vi "OFBS_displaySolution.vi"(7 "Results ListBox Ref":refnum<vi>, 8 "Stop Notifier In":refnum<notifier>, 9 "Control Refs":T1, 10 "Solution notifier":refnum<notifier>, 11 "BandGlobalOpt.lvclass":refnum<class "OptFreqBandsSearch.lvclass">) -> ()   [LabVIEW 2016, in "Optimal Frequency Bands Search.lvlib"]
doc: "Вывод текущего решения на экран. Оценка точности класификации (на тестовых данных). Обновление графиков приспособленности и точности классификации."
uses:
  GA_core/GA_tSolution progress.ctl
  OptFreqBandsSearch.lvclass
  OFBS_DataTypes.ctl
  Optimal Frequency Bands Search.lvlib
  GA_core/GeneticAlgorithm.lvlib
panel:
  # "This VI is a part of BCI Design library, http://www.ru-bci.org \nCopyright © 2020, Sotnikov Peter, All rights reserved. License: CC BY-NC 4.0"
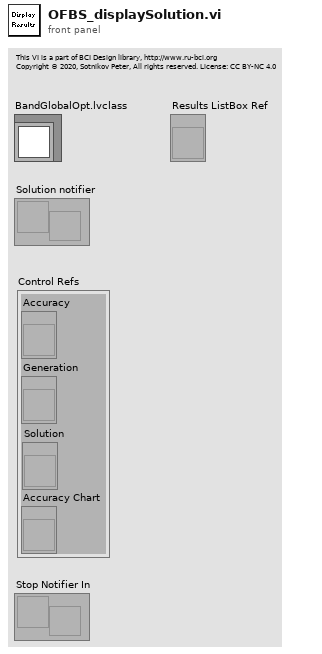
[diagram p1: front panel]
types:
  T1 = cluster{"Accuracy":refnum<vi>, "Generation":refnum<vi>, "Solution":refnum<vi>, "Accuracy Chart":refnum<vi>}
  T2 = typedef "Optimal Frequency Bands Search.lvlib/OFBS_DataTypes.ctl" = enum16{"Training Data", "Test Data", "Training Data (cross-check)", "Test Data (cross-check)"}
  T3 = typedef "Optimal Frequency Bands Search.lvlib/GeneticAlgorithm.lvlib/GA_tSolution progress.ctl" = cluster{"Solution":i32[], "Fitness":dbl, "Mutation rate":dbl, "Generation":i32}
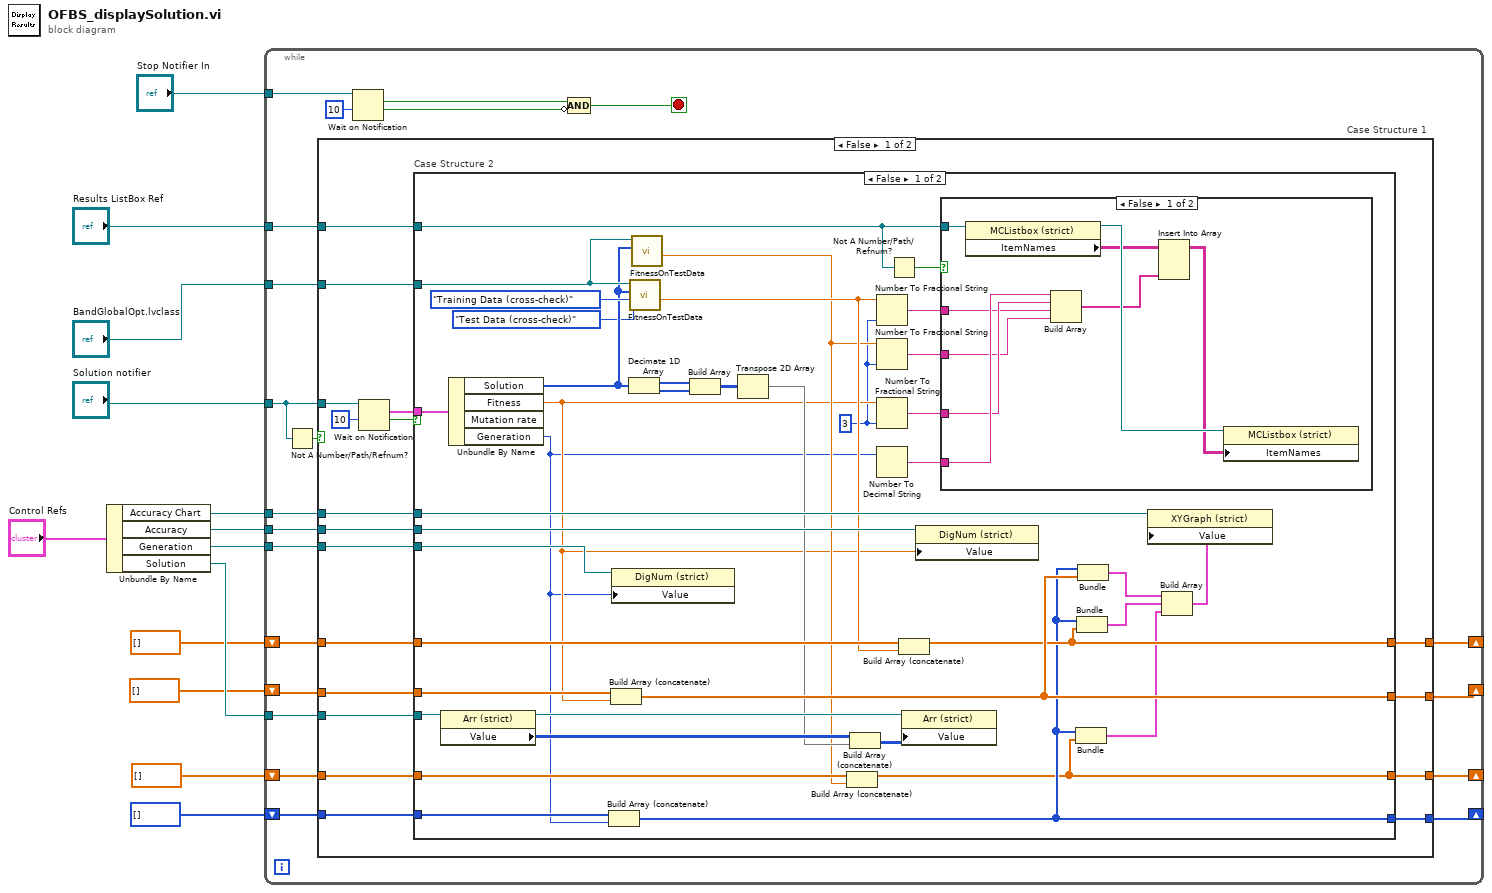
[diagram p0: block diagram]
diagram:
  n1 = Unbundle By Name("Control Refs") -> ("Accuracy Chart"=w12:refnum<vi>, "Accuracy"=w11:refnum<vi>, "Generation"=w10:refnum<vi>, "Solution"=w9:refnum<vi>)
  n2 = while {
    tunnel: "Solution notifier" -> [w33]
    tunnel: "Stop Notifier In" -> [w32]
    shift-right: [w26] -> _
    shift-left: dbl[] [] -> [w27]
    tunnel: w12 -> [w25]
    tunnel: w11 -> [w24]
    tunnel: w10 -> [w23]
    tunnel: w9 -> [w22]
    shift-right: [w20] -> _
    shift-left: i32[] [] -> [w21]
    shift-right: [w18] -> _
    shift-left: dbl[] [] -> [w19]
    tunnel: "BandGlobalOpt.lvclass" -> [w17]
    shift-right: [w15] -> _
    shift-left: dbl[] [] -> [w16]
    tunnel: "Results ListBox Ref" -> [w14]
    stop <- w28 stop-if-true
    n3 = Not A Number/Path/Refnum?(number/path/refnum=w33) -> (NaN/Path/Refnum?=w34:bool)
    n4 = case "Case Structure 1" shown="False" w34 {
      tunnel: w33 -> [w52 _]
      tunnel: w27 -> [w48 w108]
      tunnel: [w47 w108] -> w26
      tunnel: w25 -> [w46 _]
      tunnel: w24 -> [w45 _]
      tunnel: w23 -> [w44 _]
      tunnel: w22 -> [w43 _]
      tunnel: w21 -> [w42 w107]
      tunnel: [w41 w107] -> w20
      tunnel: w19 -> [w40 w106]
      tunnel: [w39 w106] -> w18
      tunnel: w17 -> [w38 _]
      tunnel: w16 -> [w37 w105]
      tunnel: [w36 w105] -> w15
      tunnel: w14 -> [w35 _]
      frame False {
        n5 = Wait on Notification(notifier=w52, timeout in ms (-1)=10) -> (notification=w50:T3, timed out?=w51:bool)  [unwired: 2 in, 2 out]
        n6 = case "Case Structure 2" shown="False" w51 {
          tunnel: w50 -> [w91 _]
          tunnel: w48 -> [w90 w104]
          tunnel: [w85 w104] -> w47
          tunnel: w46 -> [w89 _]
          tunnel: w45 -> [w88 _]
          tunnel: w44 -> [w87 _]
          tunnel: w43 -> [w79 _]
          tunnel: w42 -> [w86 w103]
          tunnel: [w70 w103] -> w41
          tunnel: w40 -> [w84 w102]
          tunnel: [w83 w102] -> w39
          tunnel: w38 -> [w66 _]
          tunnel: w37 -> [w71 w101]
          tunnel: [w69 w101] -> w36
          tunnel: w35 -> [w63 _]
          frame False {
            w57 = i16 3 ("precision (6)")
            n7 = property class="Arr (strict)"(reference=w79) -> (reference out=w78:refnum<vi>, "Value"=w75:i32[][][])  [unwired: 1 in, 1 out]
            n8 = Unbundle By Name(w91) -> ("Solution"=w65:i32[], "Fitness"=w59:dbl, "Generation"=w58:i32)  [unwired: 1 out]
            n9 = Build Array (concatenate)(w86, w58) -> (w70:i32[])
            n10 = Build Array (concatenate)(w90, w59) -> (w85:dbl[])
            n11 = property class="DigNum (strict)"(reference=w87, "Value"=w58) -> ()  [unwired: 1 in, 2 out]
            n12 = Decimate 1D Array(w65) -> (w77:i32[], w76:i32[])
            n13 = call "FitnessOnTestData.vi"("Test Data"=OFBS_DataTypes."Test Data (cross-check)", "Training Data"=OFBS_DataTypes."Training Data (cross-check)", "Phenotype"=w65, "BandGlobalOpt.lvclass"=w66) -> ("Fitness"=w61:dbl)  [unwired: 7 in]
            n14 = call "FitnessOnTestData.vi"("Phenotype"=w65, "BandGlobalOpt.lvclass"=w66) -> ("Fitness"=w60:dbl)  [unwired: 9 in]
            n15 = Build Array(w77, w76) -> (w73:i32[][])
            n16 = Transpose 2D Array(2D array=w73) -> (transposed array=w72:i32[][])
            n17 = Build Array (concatenate)(w71, w60) -> (w69:dbl[])
            n18 = Build Array (concatenate)(w75, w72) -> (w74:i32[][][])
            n19 = Number To Fractional String(number=w61, precision (6)=w57) -> (F-format string=w53:string)  [unwired: 2 in]
            n20 = Number To Fractional String(number=w60, precision (6)=w57) -> (F-format string=w54:string)  [unwired: 2 in]
            n21 = Number To Fractional String(number=w59, precision (6)=w57) -> (F-format string=w55:string)  [unwired: 2 in]
            n22 = Number To Decimal String(number=w58) -> (decimal integer string=w56:string)  [unwired: 1 in]
            n23 = Not A Number/Path/Refnum?(number/path/refnum=w63) -> (NaN/Path/Refnum?=w62:bool)
            n24 = Build Array (concatenate)(w84, w61) -> (w83:dbl[])
            n25 = property class="Arr (strict)"(reference=w78, "Value"=w74) -> ()  [unwired: 1 in, 2 out]
            n26 = property class="DigNum (strict)"(reference=w88, "Value"=w59) -> ()  [unwired: 1 in, 2 out]
            n27 = case shown="False" w62 {
              tunnel: w63 -> [w100 _]
              tunnel: w56 -> [w98 _]
              tunnel: w55 -> [w97 _]
              tunnel: w54 -> [w95 _]
              tunnel: w53 -> [w96 _]
              frame False {
                n28 = property class="MCListbox (strict)"(reference=w100) -> (reference out=w99:refnum<vi>, "ItemNames"=w94:string[][])  [unwired: 1 in, 1 out]
                n29 = Build Array(w98, w97, w96, w95) -> (w93:string[])
                n30 = Insert Into Array(array=w94, new element=w93) -> (w92:string[][])  [unwired: 2 in]
                n31 = property class="MCListbox (strict)"(reference=w99, "ItemNames"=w92) -> ()  [unwired: 1 in, 2 out]
              }
              frame True {
              }
            }
            n32 = Bundle(w70, w69) -> (w68:cluster{i32[], dbl[]})  [unwired: 1 in]
            n33 = Bundle(w70, w83) -> (w81:cluster{i32[], dbl[]})  [unwired: 1 in]
            n34 = Bundle(w70, w85) -> (w82:cluster{i32[], dbl[]})  [unwired: 1 in]
            n35 = Build Array(w82, w81, w68) -> (w80:cluster{i32[], dbl[]}[])
            n36 = property class="XYGraph (strict)"(reference=w89, "Value"=w80) -> ()  [unwired: 1 in, 2 out]
          }
          frame True {
          }
        }
      }
      frame True {
      }
    }
    n37 = Wait on Notification(notifier=w32, timeout in ms (-1)=10) -> (notification=w30:bool, timed out?=w29:bool)  [unwired: 2 in, 2 out]
    n38 = Compound Arithmetic op=AND(w30, invert w29) -> (w28:bool)
  }
